vi "Add Hardware.vi"(8 "error in (no error)":errorcluster, 9 "Chassis Settings":T18={"Chassis Settings"={"Name"="", "Master Chassis"={"Type"=enum."None", "DAQ Name"="", "clkSrc"=10280, "activeEdge"=0, "exportClk"=0, "exportClkToLine"=0, "triggerLine"=10171, "triggerSlope"=0, "startTrigger"=0, "startTriggerLine"=0}}, "DAQ Boards"=[], "FPGA Boards"=[], "CAN Boards"=[]} {"Chassis Settings"."Master Chassis"."startTriggerLine" items=["None", "PFI_0", "PFI_1", "PFI_2", "PFI_3", "PFI_4", "PFI_5", "PFI_6", "PFI_7", "PFI_8", "PFI_9", "PFI_10", "PFI_11", "PFI_12", "PFI_13", "PFI_14", "PFI_15", "RTSI_PXI_TRIG_0", "RTSI_PXI_TRIG_1", "RTSI_PXI_TRIG_2", "RTSI_PXI_TRIG_3", "RTSI_PXI_TRIG_4", "RTSI_PXI_TRIG_5", "RTSI_PXI_TRIG_6", "RTSI_PXI_TRIG_7"]; "Chassis Settings"."Master Chassis"."startTrigger" items=["aiStartTrigger", "aoStartTrigger"]; "Chassis Settings"."Master Chassis"."triggerSlope" items=["Falling"=10171, "Rising"=10280]; "Chassis Settings"."Master Chassis"."triggerLine" items=["None", "PFI_0", "PFI_1", "PFI_2", "PFI_3", "PFI_4", "PFI_5", "PFI_6", "PFI_7", "PFI_8", "PFI_9", "PFI_10", "PFI_11", "PFI_12", "PFI_13", "PFI_14", "PFI_15", "RTSI_PXI_TRIG_0", "RTSI_PXI_TRIG_1", "RTSI_PXI_TRIG_2", "RTSI_PXI_TRIG_3", "RTSI_PXI_TRIG_4", "RTSI_PXI_TRIG_5", "RTSI_PXI_TRIG_6", "RTSI_PXI_TRIG_7"]; "Chassis Settings"."Master Chassis"."exportClkToLine" items=["Default_RTSI_PXI_TRIG_0", "PFI_0", "PFI_1", "PFI_2", "PFI_3", "PFI_4", "PFI_5", "PFI_6", "PFI_7", "PFI_8", "PFI_9", "PFI_10", "PFI_11", "PFI_12", "PFI_13", "PFI_14", "PFI_15", "RTSI_PXI_TRIG_0", "RTSI_PXI_TRIG_1", "RTSI_PXI_TRIG_2", "RTSI_PXI_TRIG_3", "RTSI_PXI_TRIG_4", "RTSI_PXI_TRIG_5", "RTSI_PXI_TRIG_6", "RTSI_PXI_TRIG_7"]; "Chassis Settings"."Master Chassis"."exportClk" items=["aiSampleClock", "aoSampleClock"]; "Chassis Settings"."Master Chassis"."activeEdge" items=["Falling"=10171, "Rising"=10280]; "Chassis Settings"."Master Chassis"."clkSrc" items=["Onboard10MHzClock", "PFI_0", "PFI_1", "PFI_2", "PFI_3", "PFI_4", "PFI_5", "PFI_6", "PFI_7", "PFI_8", "PFI_9", "PFI_10", "PFI_11", "PFI_12", "PFI_13", "PFI_14", "PFI_15", "RTSI_PXI_TRIG_0", "RTSI_PXI_TRIG_1", "RTSI_PXI_TRIG_2", "RTSI_PXI_TRIG_3", "RTSI_PXI_TRIG_4", "RTSI_PXI_TRIG_5", "RTSI_PXI_TRIG_6", "RTSI_PXI_TRIG_7"]; "DAQ Boards"."Counter Settings"."Position Measurements"."ZIndexMode" items=["AHighBHigh"=10040, "AHighBLow"=10041, "ALowBHigh"=10042, "ALowBLow"=10043]; "DAQ Boards"."Counter Settings"."Position Measurements"."Decoding" items=["Decoding1X"=10090, "Decoding2X"=10091, "Decoding4X"=10092, "DecodingPulseCounting"=10313]; "DAQ Boards"."Counter Settings"."Count Measurements"."CountDirection" items=["Down"=10124, "Up"=10128, "ExternallyControlled"=10326]; "DAQ Boards"."Counter Settings"."Count Measurements"."Edge" items=["Falling"=10171, "Rising"=10280]; "DAQ Boards"."Counter Settings"."Period Measurements"."Edge" items=["Falling"=10171, "Rising"=10280]; "DAQ Boards"."Counter Settings"."Frequency Measurements"."Edge" items=["Falling"=10171, "Rising"=10280]; "DAQ Boards"."Analog Outputs"."ChannelType" items=["Voltage", "Current"]; "DAQ Boards"."Analog Inputs"."ChannelType" items=["Voltage", "Current"]; "DAQ Boards"."DAQConversionRateOption" items=["Default", "Maximum"]; "DAQ Boards"."InputConfiguration" items=["NRSE"=10078, "RSE"=10083, "Differential"=10106, "Pseudodifferential"=12529, "Default"=-1]; "CAN Boards"."Log Files"."Operation" items=["ContinueLoggingInNewFile", "StopLogging"]; "CAN Boards"."Log Files"."LimitType" items=["Footprint", "Time"]; "CAN Boards"."Log Files"."TriggerType" items=["StartLoggingOnNonZero", "StartLoggingOnZero", "EnableLoggingWhenTriggerIsZero", "EnableLoggingWhenTriggerIsNonZero"]; "CAN Boards"."Log Files"."Filter" items=["LogEntireBusTraffic", "ExcludeFrameIDs", "IncludeFrameIDs"]; "CAN Boards"."Log Files"."DataLoggingFileType" items=["TDMS", "NCL"]; "CAN Boards"."TransmitOrderType" items=["AsSubmitted", "ByIdentifier"]; "CAN Boards"."TransceiverType" items=["HS", "LS", "SW"]; "CAN Boards"."Termination" items=["Off", "On"]; "CAN Boards"."Outgoing Frames"."Phase" items=["Unchanged", "Reset"]; "CAN Boards"."Outgoing Frames"."TriggerType" items=["ChannelValueChange", "TriggerChannelNotZero", "ChannelValueChangeOrTriggerChannelNotZero"]}, 10 "Hardware":string, 11 "System Definition Ref":T19) -> (0 "error out":errorcluster, 3 "System Definition Ref":T19)   [LabVIEW 2019, in "Simple SysDef API.lvlib"]
uses:
  <userlib>/SimpleSysDef/Simple SysDef API.lvlib
  <userlib>/SimpleSysDef/_SubVIs/System Definition Reference.ctl
  NationalInstruments.VeriStand.SystemDefinitionAPI
  <userlib>/SimpleSysDef/_SubVIs/Edit Chassis_Settings.ctl
  <userlib>/SimpleSysDef/_SubVIs/Add Chassis_DAQ Master Settings.ctl
  <userlib>/SimpleSysDef/_SubVIs/Add Chassis_Type.ctl
  <userlib>/SimpleSysDef/_SubVIs/Add DAQ Hardware_Settings.ctl
  <userlib>/SimpleSysDef/_SubVIs/Add DAQ Hardware_Analog Settings.ctl
  <userlib>/SimpleSysDef/_SubVIs/Add DAQ Hardware_Digital Port Settings.ctl
  <userlib>/SimpleSysDef/_SubVIs/Add DAQ Hardware_Digital Settings.ctl
  <userlib>/SimpleSysDef/_SubVIs/Add Frequency Measurement Channels_Settings.ctl
  <userlib>/SimpleSysDef/_SubVIs/Add Count Measurement Channels_Settings.ctl
  <userlib>/SimpleSysDef/_SubVIs/Add Position Measurement Channels_Settings.ctl
  <userlib>/SimpleSysDef/_SubVIs/Add FPGA Hardware_Settings.ctl
  <userlib>/SimpleSysDef/_SubVIs/Add NI-XNET CAN Hardware_Port Settings.ctl
  <userlib>/SimpleSysDef/_SubVIs/Add NI-XNET CAN Hardware_Periodic Frame Settings.ctl
  <userlib>/SimpleSysDef/_SubVIs/Add NI-XNET CAN Hardware_Frame Settings.ctl
  <userlib>/SimpleSysDef/_SubVIs/Add NI-XNET CAN Hardware_Signal Settings.ctl
  <userlib>/SimpleSysDef/_SubVIs/Add NI-XNET CAN Hardware_Sporadic Frame Settings.ctl
  <userlib>/SimpleSysDef/_SubVIs/Add NI-XNET CAN Hardware_Add Log File_Settings.ctl
  <userlib>/SimpleSysDef/_SubVIs/Add Chassis_Settings.ctl
  <userlib>/SimpleSysDef/_SubVIs/Add Chassis.vi
  <userlib>/SimpleSysDef/_SubVIs/Add DAQ Hardware.vi
  <userlib>/SimpleSysDef/_SubVIs/Add FPGA Hardware.vi
  <userlib>/SimpleSysDef/_SubVIs/Add NI-XNET CAN Hardware.vi
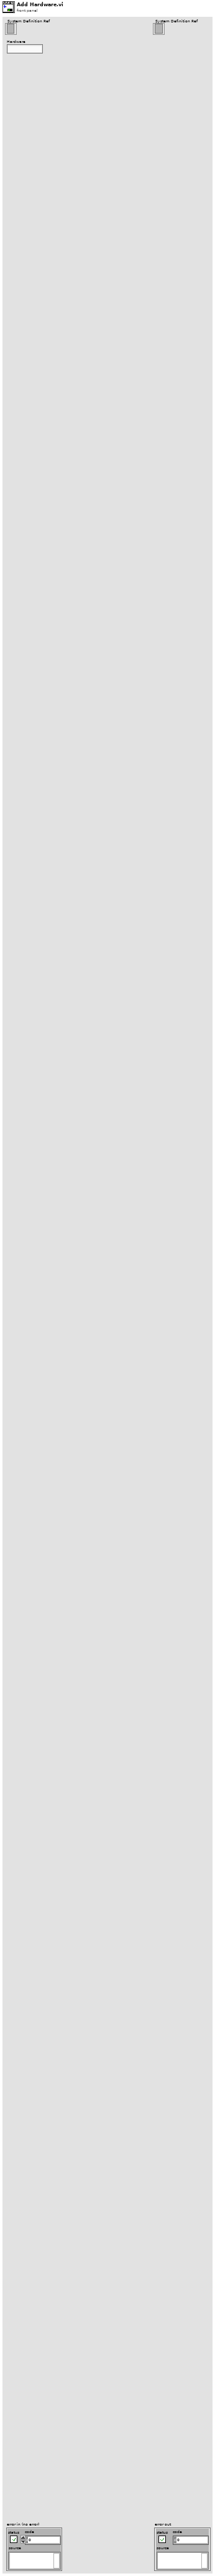
[diagram p1: front panel]
types:
  T1 = typedef "Simple SysDef API.lvlib/Edit Chassis_Settings.ctl" = cluster{"Name":string, "Master Chassis":T2}
  T2 = typedef "Simple SysDef API.lvlib/Add Chassis_DAQ Master Settings.ctl" = cluster{"Type":T3, "DAQ Name":string, "clkSrc":i32, "activeEdge":i32, "exportClk":i32, "exportClkToLine":i32, "triggerLine":i32, "triggerSlope":i32, "startTrigger":i32, "startTriggerLine":i32}
  T3 = typedef "Simple SysDef API.lvlib/Add Chassis_Type.ctl" = enum16{"None", "DAQ", "FPGA", "Timing and Sync", "Automatic"}
  T4 = typedef "Simple SysDef API.lvlib/Add DAQ Hardware_Settings.ctl" = cluster{"Name":string, "Description":string, "InputConfiguration":i32, "TurnOffHWTimedSinglePointAI":bool, "TurnOffHWTimedSinglePointAO":bool, "DAQConversionRateOption":i32, "PortWidth":u16, "Analog Inputs":T5[], "Analog Outputs":T5[], "DIO Port Settings":T6[], "Counter Settings":cluster{"Frequency Measurements":T8[], "Period Measurements":T8[], "Count Measurements":T9[], "Position Measurements":T10[]}}
  T5 = typedef "Simple SysDef API.lvlib/Add DAQ Hardware_Analog Settings.ctl" = cluster{"Name":string, "Units":string, "InitialValue":dbl, "HighLevel":dbl, "LowLevel":dbl, "Channel":u32, "ChannelType":i32, "Alias Name":string}
  T6 = typedef "Simple SysDef API.lvlib/Add DAQ Hardware_Digital Port Settings.ctl" = cluster{"portNumber":u32, "Inverted":bool, "Digital Inputs":T7[], "Digital Outputs":T7[]}
  T7 = typedef "Simple SysDef API.lvlib/Add DAQ Hardware_Digital Settings.ctl" = cluster{"Name":string, "InitialValue":bool, "DigitalLine":u32, "Alias Name":string}
  T8 = typedef "Simple SysDef API.lvlib/Add Frequency Measurement Channels_Settings.ctl" = cluster{"Name":string, "Description":string, "Units":string, "Counter":u32, "DefaultValue":dbl, "Maximum":dbl, "Minimum":dbl, "Edge":i32, "Alias Name":string}
  T9 = typedef "Simple SysDef API.lvlib/Add Count Measurement Channels_Settings.ctl" = cluster{"Name":string, "Description":string, "Units":string, "Counter":u32, "DefaultValue":dbl, "CountDirection":i32, "Edge":i32, "ResetVariable":refnum<k24>, "Alias Name":string}
  T10 = typedef "Simple SysDef API.lvlib/Add Position Measurement Channels_Settings.ctl" = cluster{"Name":string, "Description":string, "Units":string, "Counter":u32, "DefaultValue":dbl, "Decoding":i32, "ZIndexMode":i32, "Alias Name":string}
  T11 = typedef "Simple SysDef API.lvlib/Add FPGA Hardware_Settings.ctl" = cluster{"Path":path, "RIO Name":string, "Aliases":cluster{"Relative Node Path":string, "Alias Name":string}[]}
  T12 = typedef "Simple SysDef API.lvlib/Add NI-XNET CAN Hardware_Port Settings.ctl" = cluster{"Name":string, "Database Name":string, "PortNumber":u16, "ClusterName":string, "BaudRate":u32, "InlineIncoming":bool, "IncomingRate":u32, "InlineOutgoing":bool, "OutgoingRate":u32, "Termination":i32, "Echo":bool, "InputStreamQueueSize":u32, "CANBusOff":bool, "CANBusOffRate":u32, "TransceiverType":i32, "TransmitOrderType":i32, "Cyclic Frames":T13[], "Outgoing Frames":T16[], "Incoming Frames":T14[], "Log Files":T17[]}
  T13 = typedef "Simple SysDef API.lvlib/Add NI-XNET CAN Hardware_Periodic Frame Settings.ctl" = cluster{"Frame Settings":T14, "Trigger Node Path":string, "TriggerType":i32, "Disable Node Path":string}
  T14 = typedef "Simple SysDef API.lvlib/Add NI-XNET CAN Hardware_Frame Settings.ctl" = cluster{"Name":string, "ID":u32, "PayloadLength":u32, "StartTimeOffset":dbl, "Enable64Bit":bool, "Signals":T15[]}
  T15 = typedef "Simple SysDef API.lvlib/Add NI-XNET CAN Hardware_Signal Settings.ctl" = cluster{"Name":string, "Description":string, "Units":string, "DefaultValue":dbl, "Alias Name":string}
  T16 = typedef "Simple SysDef API.lvlib/Add NI-XNET CAN Hardware_Sporadic Frame Settings.ctl" = cluster{"Frame Settings":T14, "Trigger Node Path":string, "TriggerType":i32, "Disable Node Path":string, "EnableSoftwareCyclicTrigger":bool, "TransmitTime":dbl, "Phase":i32}
  T17 = typedef "Simple SysDef API.lvlib/Add NI-XNET CAN Hardware_Add Log File_Settings.ctl" = cluster{"Name":string, "Filename":string, "Destination Folder":path, "NumberOfBytesToRead":u32, "DataLoggingFileType":i32, "TDMSGroupName":string, "TDMSChannelName":string, "Filter":i32, "FrameIDs":string[], "TriggerType":i32, "LimitType":i32, "LimitValue":u32, "Operation":i32, "Retriggerable":bool, "Trigger Node Path":string}
  T18 = cluster{"Chassis Settings":T1, "DAQ Boards":T4[], "FPGA Boards":T11[], "CAN Boards":T12[]}
  T19 = typedef "Simple SysDef API.lvlib/System Definition Reference.ctl" = refnum<k24>
  T20 = typedef "Simple SysDef API.lvlib/Add Chassis_Settings.ctl" = cluster{"Name":string}
  T21 = typedef "Simple SysDef API.lvlib/Chassis Node Paths.ctl" = cluster{"Chassis":string, "DAQ":string, "Data Sharing":string, "FPGA":string, "NI-XNET CAN":string, "NI-XNET FlexRay":string, "NI-XNET LIN":string, "Timing and Sync":string}
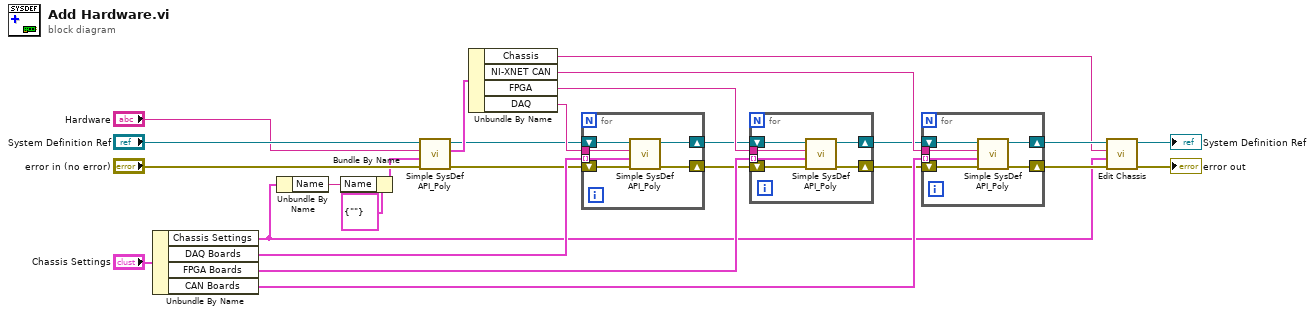
[diagram p0: block diagram]
diagram:
  n1 = Unbundle By Name("Chassis Settings") -> ("Chassis Settings"=w1:T1, "DAQ Boards"=w16:T4[], "FPGA Boards"=w22:T11[], "CAN Boards"=w26:T12[])
  n2 = Unbundle By Name(w1) -> ("Name"=w9:string)
  n3 = Bundle By Name(cluster=T20 {"Name"=""} ("Settings"), "Name"=w9) -> (w7:T20)
  n4 = call-poly <userlib>:"Simple SysDef API_Poly.vi"("error in (no error)"="error in (no error)", "Settings"=w7, "Base Node Path"="Hardware", "SysDef Ref"="System Definition Ref") -> ("error out"=w11:errorcluster, "Chassis Node Paths"=w18:T21, "SysDef Ref Out"=w12:T19)  [unwired: 5 in]
  n5 = Unbundle By Name(w18) -> ("Chassis"=w2:string, "NI-XNET CAN"=w25:string, "FPGA"=w21:string, "DAQ"=w14:string)
  n6 = for {
    tunnel: w14 -> [w29]
    tunnel: w16 -> [w28] mode=indexing
    shift-right: [w32] -> w19
    shift-left: w11 -> [w30]
    shift-right: [w31] -> w20
    shift-left: w12 -> [w27]
    n7 = call-poly <userlib>:"Simple SysDef API_Poly.vi"("error in (no error)"=w30, "Settings"=w28, "Base Node Path"=w29, "SysDef Ref"=w27) -> ("error out"=w32:errorcluster, "SysDef Ref Out"=w31:T19)  [unwired: 5 in, 1 out]
  }
  n8 = for {
    tunnel: w21 -> [w35]
    tunnel: w22 -> [w34] mode=indexing
    shift-right: [w38] -> w23
    shift-left: w19 -> [w36]
    shift-right: [w37] -> w24
    shift-left: w20 -> [w33]
    n9 = call-poly <userlib>:"Simple SysDef API_Poly.vi"("error in (no error)"=w36, "FPGA Settings"=w34, "Base Node Path"=w35, "SysDef Ref"=w33) -> ("error out"=w38:errorcluster, "SysDef Ref Out"=w37:T19)  [unwired: 5 in, 1 out]
  }
  n10 = for {
    tunnel: w25 -> [w41]
    shift-right: [w44] -> w6
    shift-left: w23 -> [w42]
    shift-right: [w43] -> w4
    shift-left: w24 -> [w40]
    tunnel: w26 -> [w39] mode=indexing
    n11 = call-poly <userlib>:"Simple SysDef API_Poly.vi"("error in (no error)"=w42, "CAN Settings"=w39, "Base Node Path"=w41, "SysDef Ref"=w40) -> ("error out"=w44:errorcluster, "SysDef Ref Out"=w43:T19)  [unwired: 5 in, 1 out]
  }
  n12 = call <userlib>:"Edit Chassis.vi"("error in (no error)"=w6, "Settings"=w1, "System Definition Node Path"=w2, "SysDef Ref"=w4) -> ("error out"=→"error out":errorcluster, "SysDef Ref Out"=→"System Definition Ref":T19)  [unwired: 5 in, 1 out]
